vi "Dashboard Main.vi"() -> ()   [LabVIEW 2012]
uses:
  <vilib>/event_ctls.llb/eventvkey.ctl
  <vilib>/Utility/miscctls.llb/LVPointTypeDef.ctl
  <vilib>/Utility/config.llb/Read Key (String).vi
  <vilib>/Utility/config.llb/Read Key (I32).vi
  <vilib>/Utility/config.llb/Write Key (String).vi
  <vilib>/Utility/config.llb/Write Key (I32).vi
  <vilib>/Utility/config.llb/NI_LVConfig.lvlib
panel:
  in  "Camera Settings":T1={"Frate Rate"=30, "Compression"=51, "Size"=1} {"Frate Rate" scale=1.0..30.0; "Size" items=["640x480", "320x240", "160x120"]}
  out "Mode":T2(ring)=enum.""
  out "Camera IP":string="0.0.0.11"
  in  "Dashboard Tab":T3(tab)
  out "GO!! GO!! GO!!":bool
  out "Driver Ready":bool
  out "Shooter Speed":T4(ring)
  out "Shooter Encoder\nDead!!":bool
  out "Shooter Good":bool
  out "Dashboard Code Verzion":string
  out "Robot Code Version":string
  out "Shooter Good":bool
  out "Shooter Speed":dbl(graph)
  out "Wheel Speed":dbl
  out "Shooter Output":dbl
  out "Shooter Speed":T4(ring)
  out "Left Encoder":dbl
  out "Right Encoder":dbl
  out "Encoder Average":dbl
  out "Left Encoder Rate":dbl
  out "Right Encoder Rate":dbl
  out "Encoder Average Rate":dbl
  out "Gyro":dbl
  out "Battery Value":dbl(slide) scale=0.0..14.0 scale format="%#_2e"
  out "Battery":sgl(graph)
  out "JS1 Z":dbl(slide) scale=-1.0..1.0 scale format="%#_2e"
  out "JS2 Z":dbl(slide) scale=-1.0..1.0 scale format="%#_2e"
  out "Joystick 1":cluster{"X":dbl, "Y":dbl}[](graph)
  out "Joystick 2":cluster{"X":dbl, "Y":dbl}[](graph)
  out "JS Buttons 1":T5
  out "JS Buttons 2":T5
  out "MotorSlide4":dbl(slide) scale=-1.0..1.0 scale format="%#_2e"
  out "MotorSlide3":dbl(slide) scale=-1.0..1.0 scale format="%#_2e"
  out "MotorSlide2":dbl(slide) scale=-1.0..1.0 scale format="%#_2e"
  in  "MotorName3":string="Front Left"
  in  "MotorName4":string="Front Right"
  in  "MotorName1":string="Rear Left"
  in  "MotorName2":string="Rear Right"
  out "MotorChart4":dbl(graph)
  out "MotorChart3":dbl(graph)
  out "MotorChart2":dbl(graph)
  out "MotorSlide1":dbl(slide) scale=-1.0..1.0 scale format="%#_2e"
  out "MotorChart1":dbl(graph)
  out "Robot IP":string="0.0.0.0"
  in  "Slider":dbl(slide) scale=0.0..100.0 scale format="%#_3g"
  in  "On/Off":bool caption="Solenoid"
  in  "Test Name":u16(ring) items=["Select the test to run...", "Example Test", "-------------------------------", "List of tests is built in robot code.", "Replace with your own automated tests."]
  in  "Test Tree":string(tree)
  in  "Motor":cluster{"Value":dbl, "Enable":bool} {"Value" scale=-1.0..1.0 scale format="%#_3g"}
  out "Progress":T6 {"Test Progress" scale=0.0..100.0}
  in  "Rev/Fwd":cluster{"Forward":bool, "Reverse":bool}
  in  "Ring":u16(ring) items=["Auto", "Fixed indoor", "Fixed outdoor 1", "Fixed outdoor 2", "Fixed fluorescent 1", "Fixed fluorescent 2", "Hold current"]
  in  "Debug Mode":bool
  in  "Listbox":i32(listbox)
  in  "Viewer":T7(tab)
  in  "Enable Processing":bool=TRUE
  out "Mbps":dbl format="%#.1g"
  in  "Enable":bool=TRUE
  in  "DB Camera Config":bool
  out "Mbps":bool
  out "fps":dbl format="%#.1g"
  out "Image Error Message":string="Timeout in Camera Communications"
  out "Camera Image":T8(plugin-control)
  out "Vision Angle":dbl
  out "Buttons 1":cluster{"1":bool, "2":bool, "3":bool}
  out "Kinect 1":cluster{"X":dbl, "Y":dbl, "Z":dbl} {"X" scale=1.0..-1.0; "Y" scale=1.0..-1.0; "Z" scale=1.0..-1.0}
  out "Buttons 2":cluster{"1":bool, "2":bool, "3":bool}
  out "Kinect 2":cluster{"X":dbl, "Y":dbl, "Z":dbl} {"X" scale=1.0..-1.0; "Y" scale=1.0..-1.0; "Z" scale=1.0..-1.0}
  out "Version":string
  out "Skeleton Picture":picture
  out "Players":i8
  out "Tree":string(tree)
  # "Drive & Motors"
  # "Robot IP:"
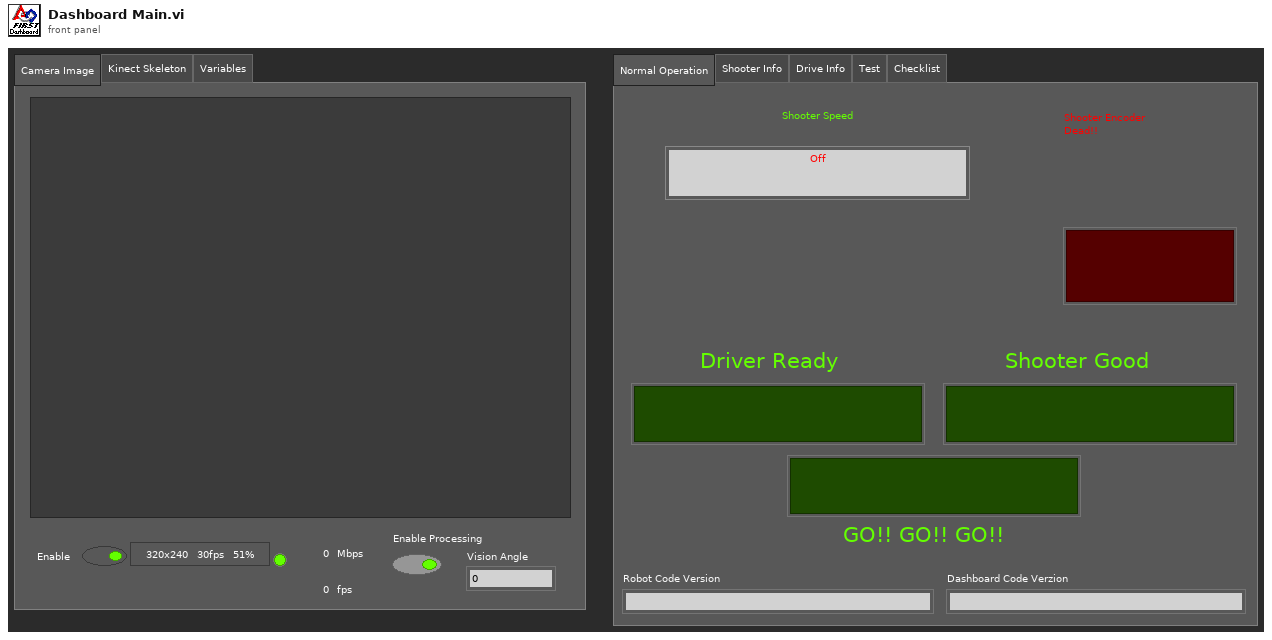
[diagram p1: front panel]
types:
  T1 = cluster{"Frate Rate":i32, "Compression":i32, "Size":u16}
  T2 = enum8{"Tele-Op Disabled", "Tele-Op Enabled", "Auto Disabled", "Auto Enabled", "Test Disabled", "Test Enabled", ""}
  T3 = enum32{"Normal Operation", "Shooter Info", "Drive Info", "Test", "Checklist"}
  T4 = enum16{"Off", "Close Pyramid 3pt", "Far Pyramid 3pt", "Feeder Shot", "UD Far 3pt Shot"}
  T5 = cluster{bool, bool, bool, bool, bool, bool, bool, bool, bool, bool, bool, bool}
  T6 = cluster{"Test Progress":u8, "Test Progress Text":string}
  T7 = enum32{"Camera Image", "Kinect Skeleton", "Variables"}
  T8 = typedef "IMAQ Image.ctl" = refnum<image>
  T9 = typedef "Image Type" = u32
  T10 = cluster{"Competition mode":bool, "Robot Link":bool, "Autonomous":bool, "Enabled":bool, "E-Stop":bool, "Simulated":bool, "TestMode":bool, "Docked Window":bool}
  T11 = cluster{"Boolean Array[0]":bool, "Boolean Array[1]":bool, "Boolean Array[2]":bool, "Boolean Array[3]":bool, "Boolean Array[4]":bool, "Boolean Array[5]":bool, "Boolean Array[6]":bool, "Boolean Array[7]":bool, "Boolean Array[8]":bool, "Boolean Array[9]":bool, "Boolean Array[10]":bool, "Boolean Array[11]":bool}
  T12 = typedef "LVPointTypeDef.ctl" = cluster{"Horizontal":i16, "Vertical":i16}
  T13 = typedef "LVRectTypeDef.ctl" = cluster{"Left":i16, "Top":i16, "Right":i16, "Bottom":i16}
  T14 = typedef "LVBoundsTypeDef.ctl" = cluster{"Width":u32, "Height":u32}
  T15 = typedef "SkeletonTrackState.ctl" = enum32{"NotTracked", "PositionOnly", "Tracked"}
  T16 = cluster{"TrackingState":u8[], "Position":cluster{"x":sgl, "y":sgl, "z":sgl}, cluster{"x":sgl, "y":sgl, "z":sgl, sgl}[], "TrackState":T15}
  T17 = cluster{cluster{"ScaledToPercentRange":dbl, "ScaledToPercentRange":dbl, "ScaledToPercentRange":dbl}, cluster{bool, bool, bool}}[]
  T18 = cluster{cluster{"ScaledToPercentRange":dbl, "ScaledToPercentRange":dbl, "ScaledToPercentRange":dbl}, cluster{bool, bool, bool}}
  T19 = cluster{"ScaledToPercentRange":dbl, "ScaledToPercentRange":dbl, "ScaledToPercentRange":dbl}
  T20 = typedef "NI_LVConfig.lvlib/Config Data RefNum.ctl" = refnum<k1>
  T21 = typedef "eventvkey.ctl" = enum16{"ASCII", "Enter", "Return", "Shift", "Ctrl", "Alt", "Cmd", "Opt", "Caps", "NumLock", "Clear", "Break", "Up", "Down", "Left", "Right", "Insert", "Delete", "Home", "End", "PageUp", "PageDown", "Escape", "Help", "Pause", "ScrollLock", "F1", "F2", "F3", "F4", "F5", "F6", "F7", "F8", "F9", "F10", "F11", "F12", "F13", "F14", "F15", "F16", "F17", "F18", "F19", "F20", "F21", "F22", "F23", "F24", "Play", "VolumeUp", "VolumeDown", "Mute", "Two Byte Char"}
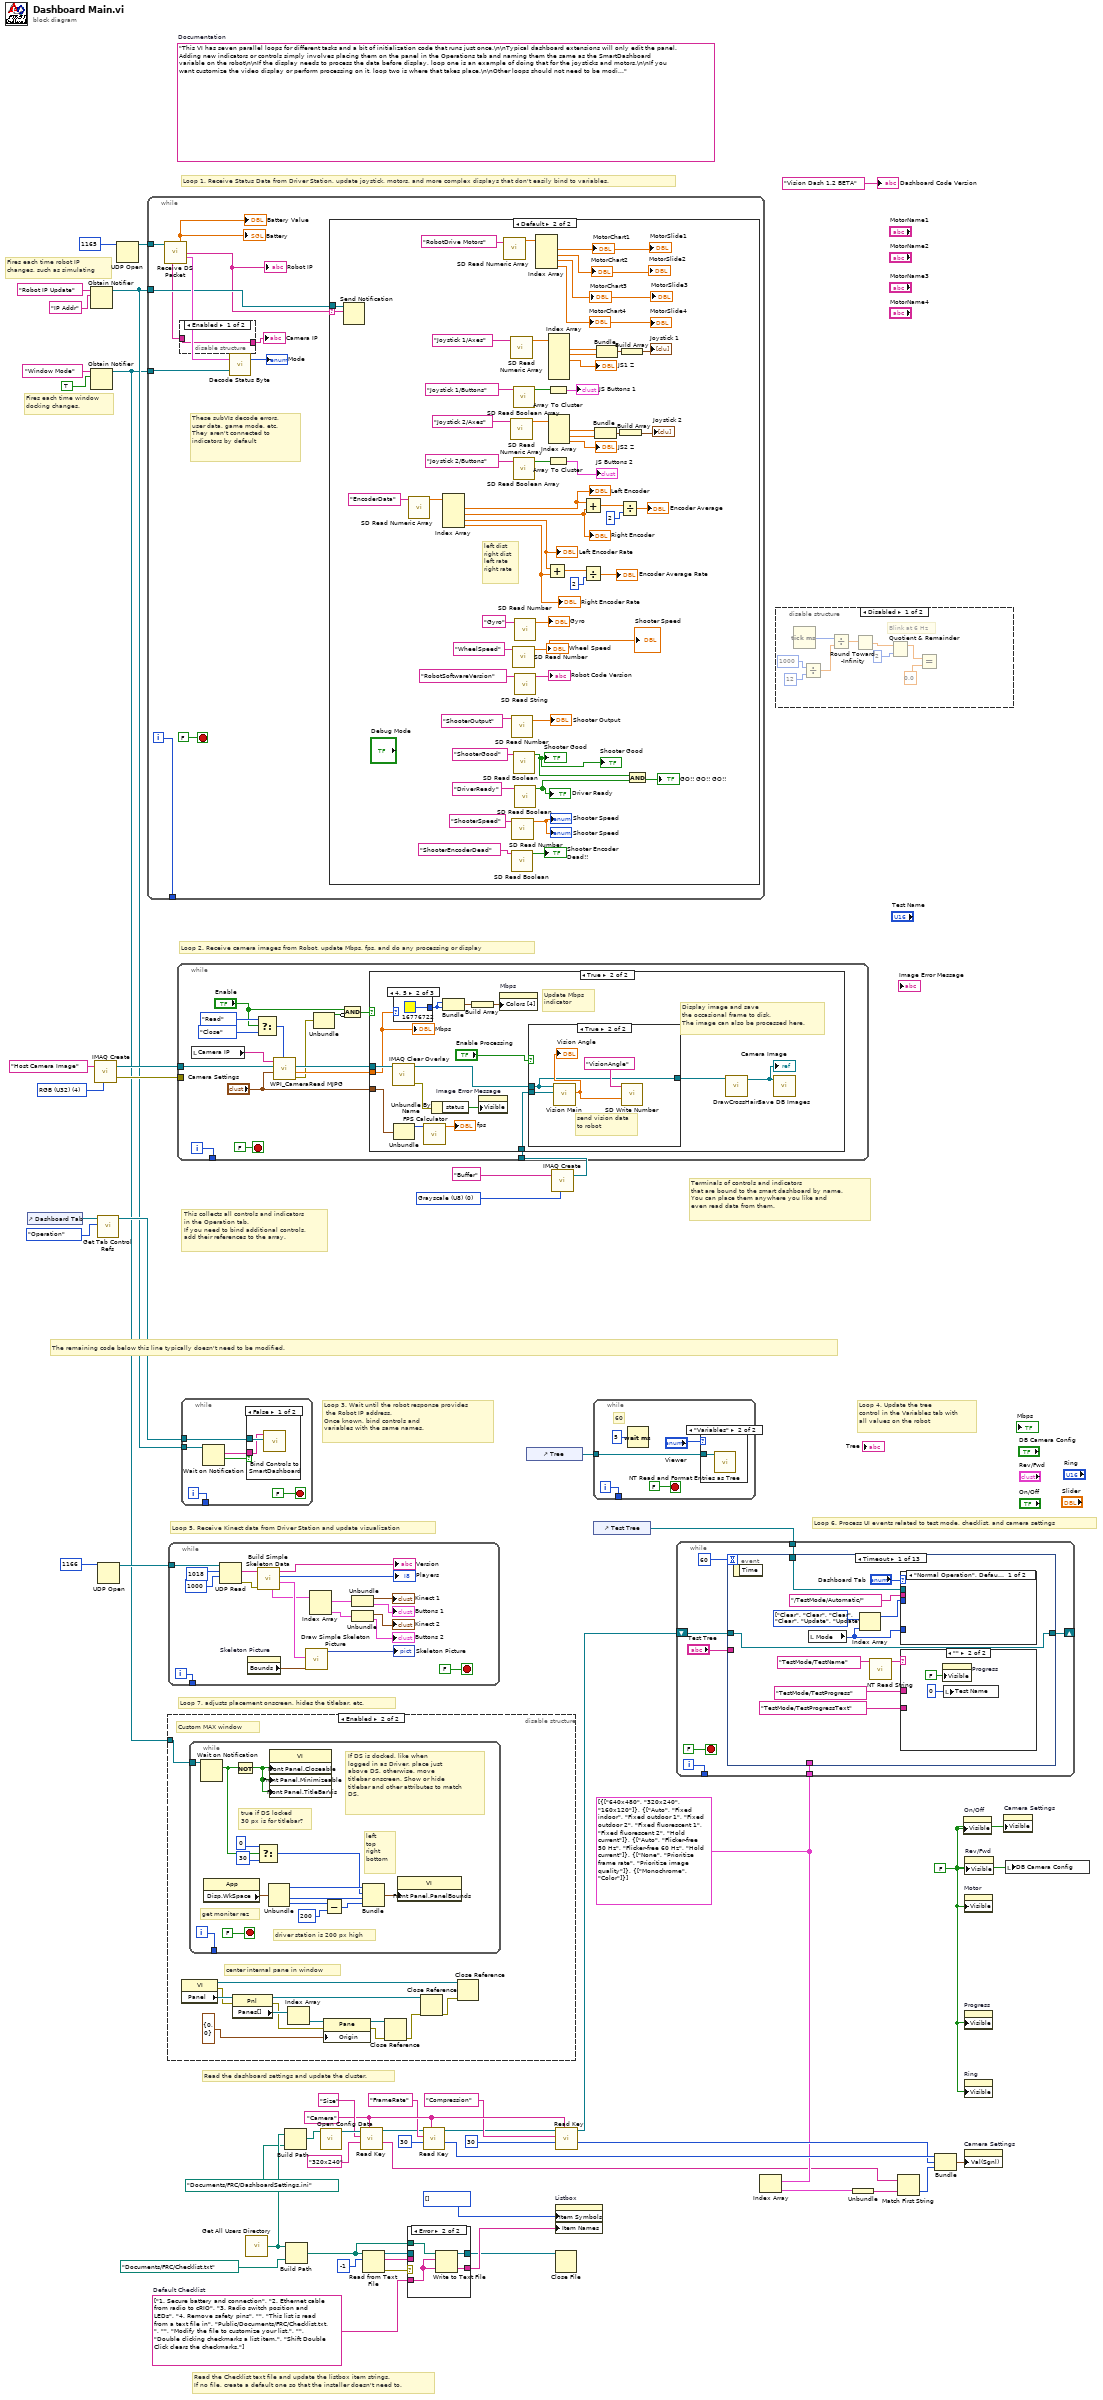
[diagram p0: block diagram]
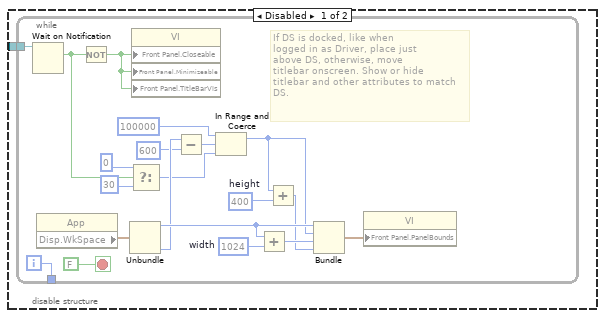
[diagram p3: hidden frame]
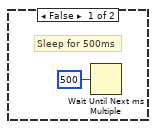
[diagram p5: hidden frame]
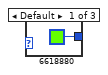
[diagram p7: hidden frame]
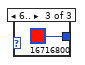
[diagram p8: hidden frame]
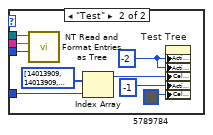
[diagram p10: hidden frame]
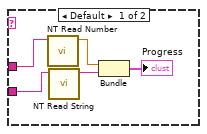
[diagram p11: hidden frame]
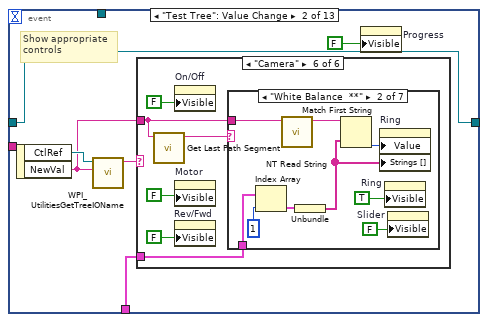
[diagram p12: hidden frame]
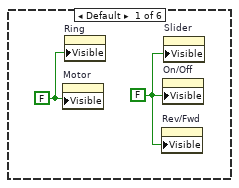
[diagram p13: hidden frame]
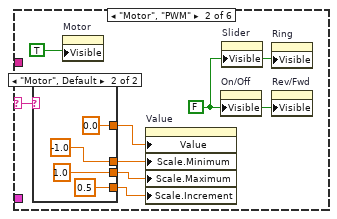
[diagram p14: hidden frame]
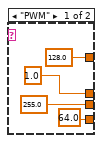
[diagram p15: hidden frame]
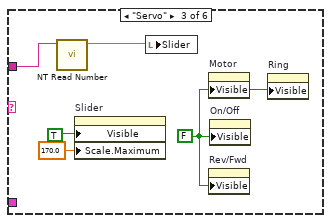
[diagram p16: hidden frame]
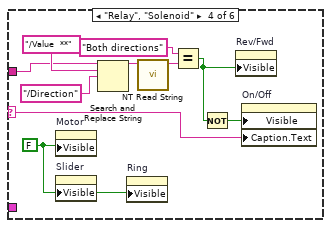
[diagram p17: hidden frame]
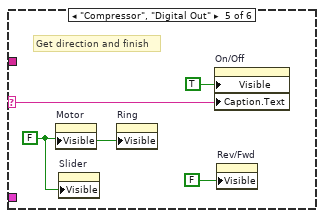
[diagram p18: hidden frame]
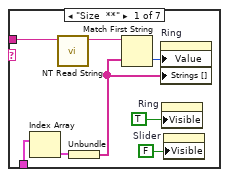
[diagram p19: hidden frame]
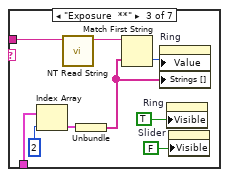
[diagram p20: hidden frame]
diagram:
  w3 = T9 0 items=["Grayscale (U8)", "Grayscale (I16)", "Grayscale (SGL)", "Complex (CSG)", "RGB (U32)", "HSL (U32)", "RGB (U64)", "Grayscale (U16)"] ("Image Type")
  w25 = "Camera"
  w17 = cluster{string[]}[] [{["640x480", "320x240", "160x120"]}, {["Auto", "Fixed indoor", "Fixed outdoor 1", "Fixed outdoor 2", "Fixed fluorescent 1", "Fixed fluorescent 2", "Hold current"]}, {["Auto", "Flicker-free 50 Hz", "Flicker-free 60 Hz", "Hold current"]}, {["None", "Prioritize frame rate", "Prioritize image quality"]}, {["Monochrome", "Color"]}]
  w33 = string[] ["1. Secure battery and connection", "2. Ethernet cable from radio to cRIO", "3. Radio switch position and LEDs", "4. Remove safety pins", "", "This list is read from a text file in", "Public/Documents/FRC/Checklist.txt.", "", "Modify the file to customize your list.", "", "Double clicking checkmarks a list item.", "Shift Double Click clears the checkmarks."]  # Default Checklist
  w31 = FALSE ("Visible")
  (unwired) "This VI has seven parallel loops for different tasks and a bit of initialization code that runs just once.\n\nTypical dashboard extensions will only edit the panel. Adding new indicators or controls simply involves placing them on the panel in the Operations tab and naming them the same as the SmartDashboard variable on the robot\n\nIf the display needs to process the data before display, loop one is an example of doing that for the joysticks and motors.\n\nIf you want customize the video display or perform processing on it, loop two is where that takes place.\n\nOther loops should not need to be modified. They are pretty standard, and document the task they perform."  # Documentation
  w54 = T9 4 items=["Grayscale (U8)", "Grayscale (I16)", "Grayscale (SGL)", "Complex (CSG)", "RGB (U32)", "HSL (U32)", "RGB (U64)"] ("Image Type")
  # "Fires each time robot IP\nchanges, such as simulating"
  # "Fires each time window\ndocking changes."
  # "Read the Checklist text file and update the listbox item strings.\nIf no file, create a default one so that the installer doesn't need to."
  # "This collects all controls and indicators\nin the Operation tab.\nIf you need to bind additional controls,\nadd their references to the array."
  # "The remaining code below this line typically doesn't need to be modified."
  # "Loop 6. Process UI events related to test mode, checklist, and camera settings"
  # "Read the dashboard settings and update the cluster."
  # "Terminals of controls and indicators\nthat are bound to the smart dashboard by name.\nYou can place them anywhere you like and\neven read data from them."
  # "Loop 4. Update the tree\ncontrol in the Variables tab with\nall values on the robot"
  # "Loop 3. Wait until the robot response provides\n the Robot IP address.\nOnce known, bind controls and\nvariables with the same names."
  # "Loop 5. Receive Kinect data from Driver Station and update visualization"
  # "Loop 7. adjusts placement onscreen, hides the titlebar, etc."
  # "Loop 1. Receive Status Data from Driver Station, update joystick, motors, and more complex displays that don't easily bind to variables."
  # "Loop 2. Receive camera images from Robot, update Mbps, fps, and do any processing or display"
  n1 = control-ref of="Dashboard Tab"() -> (w47:refnum<vi>)
  n2 = Obtain Notifier(name (unnamed)="Robot IP Update", notification data type="IP Addr" ("name (unnamed)")) -> (notifier out=w44:refnum<notifier>)  [unwired: 2 in, 2 out]
  n3 = Obtain Notifier(name (unnamed)="Window Mode", notification data type=TRUE) -> (notifier out=w37:refnum<notifier>)  [unwired: 2 in, 2 out]
  n4 = call "IMAQ Create"("Image Name"="Host Camera Image", "Image Type"=w54) -> ("New Image"=w52:T8, "error out"=w51:errorcluster)  [unwired: 2 in, 1 out]
  n5 = call <vilib>:"Get Tab Control Refs.vi"("Page Index"=enum32{"Operation", "Test"}."Operation" ("Dashboard Tab"), "TabControl in"=w47) -> ("ControlsOnPage"=w48:refnum<vi>[])  [unwired: 9 in]
  n6 = UDP Open(11:u16 1166 ("port")) -> (port=w49:refnum<k16>)  [unwired: 2 in, 4 out]
  n7 = UDP Open(11:u16 1165 ("port")) -> (port=w55:refnum<k16>)  [unwired: 2 in, 4 out]
  n8 = while {
    tunnel: w55 -> [w65]
    tunnel: w44 -> [w60]
    tunnel: w37 -> [w63]
    tunnel: [w61] -> _
    i -> [w61]
    stop <- FALSE stop-if-true
    # "These subVIs decode errors, user data, game mode, etc.\nThey aren't connected to indicators by default"
    n9 = call "Receive DS Packet.vi"("Recv Socket"=w65) -> ("Battery"=→"Battery" →"Battery Value":sgl, "Robot IP Address"=w59:string, "Status"=w66:T10, "Camera IP Address"=w57:string)  [unwired: 1 in, 10 out]
    "Robot IP" <- w59
    n10 = disable-structure shown="Enabled" {
      disable-tunnel: [w68 "10.16.76.11" ("Camera IP")] -> w58
      disable-tunnel: w57 -> [w68 _]
      frame Enabled {
      }
      frame Disabled {
      }
    }
    "Camera IP" <- w58
    n11 = call "Decode Status Byte.vi"("Window Mode Notifier"=w63, "Status"=w66) -> ("Mode"=→"Mode":T2)  [unwired: 1 out]
    n12 = case shown="Default" w59 {
      selector: w59 -> [_ w99]
      tunnel: w60 -> [_ w100]
      frame "0.0.0.0" {
        # "Robot not responding, don't poll the variables"
      }
      frame Default {
        # "left dist\nright dist\nleft rate\nright rate"
        n13 = Send Notification(notification=w99, notifier=w100) -> ()  [unwired: 1 in, 2 out]
        n14 = call <vilib>:"SD Read Numeric Array.vi"("Name"="EncoderData") -> ("Numeric Array"=w86:dbl[])  [unwired: 8 in, 2 out]
        n15 = Index Array(array=w86) -> (element #1=w85:dbl, element #2=w84:dbl, element #3=w80:dbl, element #4=w79:dbl)  [unwired: 4 in]
        "Left Encoder" <- w85
        "Right Encoder" <- w84
        "Left Encoder Rate" <- w80
        "Right Encoder Rate" <- w79
        n16 = call <vilib>:"SD Read Numeric Array.vi"("Name"="RobotDrive Motors") -> ("Numeric Array"=w123:dbl[])  [unwired: 8 in, 2 out]
        n17 = call <vilib>:"SD Read Numeric Array.vi"("Name"="Joystick 1/Axes") -> ("Numeric Array"=w116:dbl[])  [unwired: 8 in, 2 out]
        n18 = call <vilib>:"SD Read Numeric Array.vi"("Name"="Joystick 2/Axes") -> ("Numeric Array"=w110:dbl[])  [unwired: 8 in, 2 out]
        n19 = call <vilib>:"SD Read Number.vi"("Name"="ShooterOutput") -> ("Numeric"=→"Shooter Output":dbl)  [unwired: 8 in, 2 out]
        n20 = call <vilib>:"SD Read Boolean.vi"("Name"="ShooterEncoderDead") -> ("Boolean"=→"Shooter Encoder\nDead!!":bool)  [unwired: 8 in, 2 out]
        n21 = call <vilib>:"SD Read Number.vi"("Name"="ShooterSpeed") -> ("Numeric"=→"Shooter Speed" →"Shooter Speed":dbl)  [unwired: 8 in, 2 out]
        n22 = call <vilib>:"SD Read Number.vi"("Name"="WheelSpeed") -> ("Numeric"=→"Wheel Speed" →"Shooter Speed":dbl)  [unwired: 8 in, 2 out]
        n23 = call <vilib>:"SD Read Boolean Array.vi"("Name"="Joystick 1/Buttons") -> ("Boolean Array"=w118:bool[])  [unwired: 8 in, 2 out]
        n24 = call <vilib>:"SD Read Boolean Array.vi"("Name"="Joystick 2/Buttons") -> ("Boolean Array"=w109:bool[])  [unwired: 8 in, 2 out]
        n25 = call <vilib>:"SD Read Boolean.vi"("Name"="ShooterGood") -> ("Boolean"=w73:bool)  [unwired: 8 in, 2 out]
        "Shooter Good" <- w73
        "Shooter Good" <- w73
        n26 = call <vilib>:"SD Read Number.vi"("Name"="Gyro") -> ("Numeric"=→"Gyro":dbl)  [unwired: 8 in, 2 out]
        n27 = call <vilib>:"SD Read String.vi"("Name"="RobotSoftwareVersion") -> ("String"=→"Robot Code Version":string)  [unwired: 8 in, 2 out]
        n28 = call <vilib>:"SD Read Boolean.vi"("Name"="DriverReady") -> ("Boolean"=w72:bool)  [unwired: 8 in, 2 out]
        "Driver Ready" <- w72
        n29 = Index Array(array=w123) -> (element #1=→"MotorChart1" →"MotorSlide1":dbl, element #2=→"MotorSlide2" →"MotorChart2":dbl, element #3=→"MotorChart3" →"MotorSlide3":dbl, element #4=→"MotorChart4" →"MotorSlide4":dbl)  [unwired: 4 in]
        n30 = Add(x=w80, y=w79) -> (x+y=w81:dbl)
        n31 = Array To Cluster(array=w118) -> (cluster=→"JS Buttons 1":T11)
        n32 = Array To Cluster(array=w109) -> (cluster=→"JS Buttons 2":T11)
        n33 = Index Array(array=w116) -> (element #1=w113:dbl, element #2=w114:dbl, element #3=→"JS1 Z":dbl)  [unwired: 6 in, 3 out]
        n34 = Index Array(array=w110) -> (element #1=w105:dbl, element #2=w104:dbl, element #3=→"JS2 Z":dbl)  [unwired: 3 in]
        n35 = Add(x=w85, y=w84) -> (x+y=w95:dbl)
        n36 = Divide(x=w81, y=2) -> (x/y=→"Encoder Average Rate":dbl)
        n37 = Bundle("Numeric"=w105, "Numeric"=w104) -> (w106:cluster{"Numeric":dbl, "Numeric":dbl})  [unwired: 1 in]
        n38 = Bundle("Numeric"=w113, "Numeric"=w114) -> (w112:cluster{"Numeric":dbl, "Numeric":dbl})  [unwired: 1 in]
        n39 = Divide(x=w95, y=2) -> (x/y=→"Encoder Average":dbl)
        n40 = Build Array(w106) -> (→"Joystick 2":cluster{"Numeric":dbl, "Numeric":dbl}[])
        n41 = Build Array(w112) -> (→"Joystick 1":cluster{"Numeric":dbl, "Numeric":dbl}[])
        n42 = And(x=w73, y=w72) -> (x .and. y?=→"GO!! GO!! GO!!":bool)
      }
    }
  }
  n43 = disable-structure shown="Enabled" {
    disable-tunnel: w37 -> [w127 w160]
    frame Disabled {
      n44 = while {
        tunnel: w127 -> [w146]
        tunnel: [w144] -> _
        i -> [w144]
        stop <- FALSE stop-if-true
        w136 = 1024  # width
        w139 = 400  # height
        # "If DS is docked, like when\nlogged in as Driver, place just\nabove DS, otherwise, move\ntitlebar onscreen. Show or hide\ntitlebar and other attributes to match\nDS."
        n45 = Wait on Notification(notifier=w146) -> (notification=w131:bool)  [unwired: 3 in, 3 out]
        n46 = property class="App"() -> ("Disp.WkSpace"=w142:T13)  [unwired: 2 in, 2 out]
        n47 = Not(x=w131) -> (.not. x?=w145:bool)
        n48 = Unbundle(w142) -> ("Left"=w140:i16, "Bottom"=w137:i16)  [unwired: 2 out]
        n49 = Select(t=0, s=w131, f=30) -> (s? t:f=w130:i32)
        n50 = property class="VI"("Front Panel.Closeable"=w145, "Front Panel.Minimizeable"=w145, "Front Panel.TitleBarVis"=w145) -> ()  [unwired: 2 in, 2 out]
        n51 = Subtract(x=w137, y=600) -> (x-y=w134:i32)
        n52 = In Range and Coerce(upper limit=100000, x=w134, lower limit=w130) -> (coerced(x)=w128:i32)  [unwired: 1 out]
        n53 = Add(x=w140, y=w136) -> (x+y=w141:i32)
        n54 = Add(x=w128, y=w139) -> (x+y=w138:i32)
        n55 = Bundle("Left"=w140, w128, w141, w138) -> (w143:cluster{"Left":i16, i32, i32, i32})  [unwired: 1 out]
        n56 = property class="VI"("Front Panel.PanelBounds"=w143) -> ()  [unwired: 2 in, 2 out]
      }
    }
    frame Enabled {
      # "center internal pane in window"
      # "Custom MAX window"
      n57 = property class="VI"() -> (reference out=w153:refnum<vi>, error out=w152:errorcluster, "Panel"=w159:refnum<vi>)  [unwired: 2 in]
      n58 = while {
        tunnel: w160 -> [w174]
        tunnel: [w172] -> _
        i -> [w172]
        stop <- FALSE stop-if-true
        # "driver station is 200 px high"
        # "true if DS locked\n30 px is for titlebar?"
        # "left\ntop\nright\nbottom"
        # "get moniter rez"
        # "If DS is docked, like when\nlogged in as Driver, place just\nabove DS, otherwise, move\ntitlebar onscreen. Show or hide\ntitlebar and other attributes to match\nDS."
        n59 = Wait on Notification(notifier=w174) -> (notification=w166:bool)  [unwired: 3 in, 3 out]
        n60 = property class="App"() -> ("Disp.WkSpace"=w170:T13)  [unwired: 2 in, 2 out]
        n61 = Not(x=w166) -> (.not. x?=w173:bool)
        n62 = Select(t=0, s=w166, f=30) -> (s? t:f=w164:i32)
        n63 = Unbundle(w170) -> ("Left"=w169:i16, "Right"=w165:i16, "Bottom"=w162:i16)  [unwired: 1 out]
        n64 = property class="VI"("Front Panel.Closeable"=w173, "Front Panel.Minimizeable"=w173, "Front Panel.TitleBarVis"=w173) -> ()  [unwired: 2 in, 2 out]
        n65 = Subtract(x=w162, y=i16 200) -> (x-y=w163:i16)
        n66 = Bundle("Left"=w169, w164, "Right"=w165, w163) -> (w171:cluster{"Left":i16, i32, "Right":i16, i16})  [unwired: 1 out]
        n67 = property class="VI"("Front Panel.PanelBounds"=w171) -> ()  [unwired: 2 in, 2 out]
      }
      n68 = property class="Pnl"(reference=w159, error in=w152) -> (reference out=w154:refnum<vi>, error out=w151:errorcluster, "Panes[]"=w158:refnum<vi>[])
      n69 = Index Array(array=w158) -> (element=w157:refnum<vi>)  [unwired: 1 in]
      n70 = property class="Pane"(reference=w157, error in=w151, "Origin"=T12 {"Horizontal"=0, "Vertical"=0}) -> (reference out=w155:refnum<vi>, error out=w150:errorcluster)
      n71 = Close Reference(reference=w155, error in (no error)=w150) -> (error out=w149:errorcluster)
      n72 = Close Reference(reference=w154, error in (no error)=w149) -> (error out=w148:errorcluster)
      n73 = Close Reference(reference=w153, error in (no error)=w148) -> ()  [unwired: 1 out]
    }
  }
  n74 = while {
    tunnel: w49 -> [w192]
    tunnel: [w177] -> _
    i -> [w177]
    stop <- FALSE stop-if-true
    n75 = UDP Read(connection ID=w192, max size (548)=1018 ("bytes to read"), timeout ms (25000)=1000) -> (data out=w186:string, error out=w176:errorcluster)  [unwired: 1 in, 3 out]
    n76 = property on="Skeleton Picture" class="Pict"() -> ("Bounds"=w188:T14)  [unwired: 2 in, 2 out]
    n77 = call "Build Simple Skeleton Data.vi"("error in (no error)"=w176, "data in"=w186) -> ("Skeleton Data"=w187:T16, "NumPlayers"=→"Players":i8, "Version String"=→"Version":string, "Simple Joystick Info"=w184:T17)  [unwired: 5 in, 1 out]
    n78 = call "Draw Simple Skeleton Picture.vi"("Bounds"=w188, "Simple Skeleton"=w187) -> ("new picture out"=→"Skeleton Picture":picture)  [unwired: 9 in]
    n79 = Index Array(array=w184) -> (element #1=w183:T18, element #2=w182:T18)  [unwired: 2 in]
    n80 = Unbundle(w183) -> (→"Kinect 1":T19, →"Buttons 1":cluster{bool, bool, bool})
    n81 = Unbundle(w182) -> (→"Kinect 2":T19, →"Buttons 2":cluster{bool, bool, bool})
  }
  n82 = while {
    tunnel: w48 -> [w200]
    tunnel: w44 -> [w197]
    tunnel: [w195] -> _
    i -> [w195]
    stop <- FALSE stop-if-true
    n83 = Wait on Notification(notifier=w197) -> (notification=w196:string, timed out?=w198:bool)  [unwired: 3 in, 2 out]
    n84 = case shown="False" w198 {
      tunnel: w200 -> [w202 _]
      tunnel: w196 -> [w201 _]
      frame False {
        n85 = call <vilib>:"Bind Controls to SmartDashboard.vi"("Bound Control Refs"=w202, "Server IP Address"=w201) -> ()  [unwired: 10 in]
      }
      frame True {
      }
    }
  }
  n86 = call "Get All Users Directory.vi"() -> ("All User Path"=w30:path)
  n87 = Build Path(base path=w30, name or relative path=path "Documents/FRC/DashboardSettings.ini") -> (appended path=w29:path)
  n88 = Build Path(base path=w30, name or relative path=path "Documents/FRC/Checklist.txt") -> (appended path=w34:path)
  n89 = call <vilib>:"Open Config Data.vi"("configuration file path"=w29) -> ("refnum"=w28:T20)  [unwired: 8 in, 2 out]
  n90 = call-poly <vilib>:"Read Key.vi"("section"=w25, "default value"="320x240", "key"="Size", "refnum"=w28) -> ("value"=w15:string, "refnum out"=w10:T20)  [unwired: 2 in, 4 out]
  n91 = Read from Text File(file (use dialog)=w34, count=-1 ("timeout ms (25000)")) -> (refnum out=w12:refnum<file>, text=w35:string[], error out=w36:errorcluster)  [unwired: 2 in, 1 out]
  n92 = case shown="Error" w36 {
    tunnel: w35 -> [w204 _]
    tunnel: [w204 w206] -> w32
    tunnel: w33 -> [_ w206]
    tunnel: w34 -> [_ w207]
    tunnel: [w203 w205] -> w11
    tunnel: w12 -> [w203 _]
    frame No Error {
    }
    frame Error {
      n93 = Write to Text File(file (use dialog)=w207, text=w206) -> (refnum out=w205:refnum<file>)  [unwired: 2 in, 2 out]
    }
  }
  n94 = call-poly <vilib>:"Read Key.vi"("section"=w25, "default value"=30, "key"="FrameRate", "refnum"=w10) -> ("value"=w20:i32, "refnum out"=w9:T20)  [unwired: 1 in, 5 out]
  n95 = control-ref of="Tree"() -> (w6:refnum<vi>)
  n96 = call "IMAQ Create"("Image Name"="Buffer", "Image Type"=w3) -> ("New Image"=w2:T8)  [unwired: 3 in, 1 out]
  n97 = while {
    tunnel: w52 -> [w218]
    tunnel: w51 -> [_]
    tunnel: [w221] -> _
    tunnel: w2 -> [w208]
    i -> [w221]
    stop <- FALSE stop-if-true
    n98 = local read "Camera IP"() -> (w220:string)
    n99 = Select(t=enum16{"Read", "Reopen", "Close"}."Read" ("Operation"), s="Enable", f=enum16{"Read", "Reopen", "Close"}."Close" ("Operation")) -> (s? t:f=w213:enum16{"Read", "Reopen", "Close"})
    n100 = call <vilib>:"WPI_CameraRead MJPG.vi"("Operation"=w213, "Camera Settings"="Camera Settings", "Image"=w218, "address"=w220) -> ("error out"=w212:errorcluster, "Bandwidth (kbps)"=w216:dbl, "Image Out"=w217:T8)  [unwired: 5 in]
    n101 = Unbundle(w212) -> ("status"=w210:bool)  [unwired: 2 out]
    n102 = Compound Arithmetic op=AND("Enable", invert w210) -> (w209:bool)
    n103 = case shown="True" w209 {
      tunnel: "Camera Settings" -> [_ w230]
      tunnel: w217 -> [_ w233]
      tunnel: w216 -> [_ w232]
      tunnel: w208 -> [_ w228]
      frame False {
        # "Sleep for 500ms"
        n104 = Wait Until Next ms Multiple(millisecond multiple=u32 500) -> ()  [unwired: 1 out]
      }
      frame True {
        # "Display image and save\nthe occasional frame to disk.\nThe image can also be processed here."
        # "Update Mbps\nindicator"
        n105 = call "IMAQ Clear Overlay"("Image"=w233) -> ("error out"=w237:errorcluster, "Image Out"=w226:T8)  [unwired: 2 in, 7 out]
        n106 = case shown="4, 5" w232 {
          tunnel: [u32 6618880 ("Color Box") u32 16776722 ("Color Box") u32 16716800 ("Color Box")] -> w234
          frame Default {
          }
          frame 4, 5 {
          }
          frame 6.. {
          }
        }
        n107 = Unbundle(w230) -> ("Frate Rate"=w229:i32)  [unwired: 2 out]
        n108 = call "FPS Calculator.vi"("Average Count"=w229) -> ("fps"=→"fps":dbl)  [unwired: 10 in]
        n109 = Unbundle By Name(w237) -> ("status"=w238:bool)
        n110 = Bundle("Color Box"=w234, "Color Box"=w234) -> (w236:cluster{"Color Box":u32, "Color Box":u32})  [unwired: 1 out]
        n111 = Build Array(w236) -> (w235:cluster{"Color Box":u32, "Color Box":u32}[])
        n112 = property on="Image Error Message" class="Str"("Visible"=w238) -> ()  [unwired: 2 in, 2 out]
        n113 = property on="Mbps" class="Bool (strict)"("Colors [4]"=w235) -> ()  [unwired: 2 in, 2 out]
        n114 = case shown="True" "Enable Processing" {
          tunnel: w228 -> [_ w243]
          tunnel: w226 -> [w239 w240]
          tunnel: [w239 w240] -> w225
          frame False {
          }
          frame True {
            # "send vision data\nto robot"
            n115 = call "Vision Main.vi"("Frame Buffer"=w243, "Camera Image"=w240) -> ("Chosen Target Angle"=w241:dbl)  [unwired: 8 in, 1 out]
            "Vision Angle" <- w241
            n116 = call <vilib>:"SD Write Number.vi"("Numeric"=w241, "Name"="VisionAngle") -> ()  [unwired: 8 in, 2 out]
          }
        }
        n117 = call "DrawCrossHairs.vi"("Image In"=w225) -> ("Image Out"=w227:T8)  [unwired: 10 in]
        "Camera Image" <- w227
        n118 = call "Save DB Images.vi"("Image"=w227) -> ()  [unwired: 2 in, 1 out]
        "Mbps" <- w232
      }
    }
  }
  n119 = property on="Listbox" class="LstBox (strict)"("Item Symbols"=i32[] [], "Item Names"=w32) -> ()  [unwired: 2 in, 2 out]
  n120 = Close File(refnum=w11) -> ()  [unwired: 1 in, 2 out]
  n121 = call-poly <vilib>:"Read Key.vi"("section"=w25, "default value"=30, "key"="Compression", "refnum"=w9) -> ("value"=w19:i32, "refnum out"=w7:T20)  [unwired: 1 in, 5 out]
  n122 = while {
    tunnel: [w248] -> _
    tunnel: w6 -> [w247]
    i -> [w248]
    stop <- FALSE stop-if-true
    # "60"
    n123 = Wait (ms)(milliseconds to wait=u32 5) -> ()  [unwired: 1 out]
    n124 = case shown="\"Variables\"" "Viewer" {
      tunnel: w247 -> [_ w252]
      frame Default {
      }
      frame "Variables" {
        n125 = call <vilib>:"NT Read and Format Entries as Tree.vi"("Tree Refnum"=w252) -> ()  [unwired: 9 in, 2 out]
      }
    }
  }
  n126 = control-ref of="Test Tree"() -> (w5:refnum<vi>)
  n127 = while {
    tunnel: w17 -> [w257]
    shift-right: [w256] -> _
    shift-left: w7 -> [w255]
    tunnel: [w254] -> _
    tunnel: w5 -> [w253]
    i -> [w254]
    stop <- FALSE stop-if-true
    n128 = event shown="[0] Timeout" {
      selector: _ -> [_ _ _ _ _ _ _ _ _ _ _ _ _]
      dyn-events: _ -> [_ _ _ _ _ _ _ _ _ _ _ _ _]
      timeout: u32 60 ("milliseconds to wait") -> [_ _ _ _ _ _ _ _ _ _ _ _ _]
      tunnel: w253 -> [w267 _ _ _ _ _ _ _ _ _ _ _ _]
      tunnel: "Test Tree" -> [_ _ _ _ _ _ _ _ w461 w469 w471 w475 w483]
      tunnel: w257 -> [_ w289 _ _ _ _ w425 w455 _ _ _ _ _]
      tunnel: [w261 w288 _ w391 w399 w411 w424 w448 w460 w467 w470 w474 w482] -> w256
      tunnel: w255 -> [w261 w288 _ w391 w399 w411 w423 w448 w460 w467 w470 w474 w482]
      event Timeout {
        w266 = enum16{"Update", "Clear"}[] [enum."Clear", enum."Clear", enum."Clear", enum."Clear", enum."Update", enum."Update", enum."Clear"] items=["Update", "Clear"]
        n129 = event-data() -> ()  [unwired: 1 in, 1 out]
        n130 = local read "Mode"() -> (w264:T2)
        n131 = Index Array(array=w266, index=w264) -> (element=w265:enum16{"Update", "Clear"})
        n132 = call <vilib>:"NT Read String.vi"("Name"="TestMode/TestName") -> ("String"=w270:string)  [unwired: 9 in, 1 out]
        n133 = case shown="\"Normal Operation\", Default" "Dashboard Tab" {
          tunnel: w267 -> [_ w280]
          tunnel: "/TestMode/Automatic/" ("Name Pattern") -> [_ w279]
          tunnel: w265 -> [_ w278]
          tunnel: w264 -> [_ w276]
          frame "Normal Operation", Default {
          }
          frame "Test" {
            w275 = -2 ("Active Item:Row Number")
            n134 = call <vilib>:"NT Read and Format Entries as Tree.vi"("Operation"=w278, "Name Pattern"=w279, "Tree Refnum"=w280) -> ()  [unwired: 7 in, 2 out]
            n135 = Index Array(array=u32[] [14013909, 14013909, 14013909, 14013909, 14013909, 16777215, 14013909], index=w276) -> (element=w274:u32)
            n136 = property on="Test Tree" class="Tree (strict)"("Active Item Row Number"=w275, "ActiveColNum"=w275, "CellBG"=w274, "Active Item Row Number"=-1 ("Active Item:Row Number"), "CellBG"=u32 5789784 ("Color Box")) -> ()  [unwired: 2 in, 2 out]
          }
        }
        n137 = case shown="\"\"" w270 {
          tunnel: "TestMode/TestProgress" ("Name") -> [w282 _]
          tunnel: "TestMode/TestProgressText" ("Name") -> [w281 _]
          frame Default {
            n138 = call <vilib>:"NT Read Number.vi"("Name"=w282) -> ("Numeric"=w283:dbl)  [unwired: 9 in, 1 out]
            n139 = call <vilib>:"NT Read String.vi"("Name"=w281) -> ("String"=w284:string)  [unwired: 9 in, 1 out]
            n140 = Bundle("Numeric"=w283, "String"=w284) -> (→"Progress":cluster{"Numeric":dbl, "String":string})  [unwired: 1 in]
          }
          frame "" {
            n141 = property on="Progress" class="Clust (strict)"("Visible"=FALSE) -> ()  [unwired: 2 in, 2 out]
            n142 = local write "Test Name"(u16 0) -> ()
          }
        }
      }
      event "Test Tree": Value Change {
        # "Show appropriate\ncontrols"
        n143 = event-data() -> ("CtlRef"=w292:refnum<vi>, "NewVal"=w290:string)  [unwired: 1 in]
        n144 = call <vilib>:"WPI_UtilitiesGetTreeIOName.vi"("NewVal"=w290, "TreeControl in"=w292) -> ("I/O Name"=w293:string)  [unwired: 9 in]
        n145 = case shown="\"Camera\"" w293 {
          selector: w293 -> [_ w300 _ w318 w327 _]
          tunnel: w290 -> [_ _ w315 w317 _ w334]
          tunnel: w289 -> [_ _ _ _ _ w333]
          frame Default {
            w295 = FALSE ("Visible")
            w294 = FALSE ("Visible")
            n146 = property on="Motor" class="Clust (strict)"("Visible"=w294) -> ()  [unwired: 2 in, 2 out]
            n147 = property on="Ring" class="Ring (strict)"("Visible"=w294) -> ()  [unwired: 2 in, 2 out]
            n148 = property on="Rev/Fwd" class="Clust (strict)"("Visible"=w295) -> ()  [unwired: 2 in, 2 out]
            n149 = property on="On/Off" class="Bool (strict)"("Visible"=w295) -> ()  [unwired: 2 in, 2 out]
            n150 = property on="Slider" class="Slide (strict)"("Visible"=w295) -> ()  [unwired: 2 in, 2 out]
          }
          frame "Motor", "PWM" {
            w301 = FALSE ("Visible")
            n151 = case shown="\"Motor\", Default" w300 {
              tunnel: [1.0 ("Value") -1.0 ("Value")] -> w299
              tunnel: [255.0 ("Value") 1.0 ("Value")] -> w298
              tunnel: [128.0 ("Value") 0.0 ("Value")] -> w297
              tunnel: [64.0 ("Value") 0.5 ("Value")] -> w296
              frame "PWM" {
              }
              frame "Motor", Default {
              }
            }
            n152 = property on="Motor" class="Clust (strict)"("Visible"=TRUE) -> ()  [unwired: 2 in, 2 out]
            n153 = property on="Value" class="Slide (strict)"("Value"=w297, "Scale.Minimum"=w299, "Scale.Maximum"=w298, "Scale.Increment"=w296) -> ()  [unwired: 2 in, 2 out]
            n154 = property on="On/Off" class="Bool (strict)"("Visible"=w301) -> ()  [unwired: 2 in, 2 out]
            n155 = property on="Slider" class="Slide (strict)"("Visible"=w301) -> ()  [unwired: 2 in, 2 out]
            n156 = property on="Ring" class="Ring (strict)"("Visible"=w301) -> ()  [unwired: 2 in, 2 out]
            n157 = property on="Rev/Fwd" class="Clust (strict)"("Visible"=w301) -> ()  [unwired: 2 in, 2 out]
          }
          frame "Servo" {
            w313 = FALSE ("Visible")
            n158 = call <vilib>:"NT Read Number.vi"("Name"=w315) -> ("Numeric"=w314:dbl)  [unwired: 9 in, 1 out]
            n159 = property on="Slider" class="Slide (strict)"("Visible"=TRUE, "Scale.Maximum"=170.0 ("Scale.Range:Maximum")) -> ()  [unwired: 2 in, 2 out]
            n160 = local write "Slider"(w314) -> ()
            n161 = property on="Motor" class="Clust (strict)"("Visible"=w313) -> ()  [unwired: 2 in, 2 out]
            n162 = property on="Rev/Fwd" class="Clust (strict)"("Visible"=w313) -> ()  [unwired: 2 in, 2 out]
            n163 = property on="On/Off" class="Bool (strict)"("Visible"=w313) -> ()  [unwired: 2 in, 2 out]
            n164 = property on="Ring" class="Ring (strict)"("Visible"=w313) -> ()  [unwired: 2 in, 2 out]
          }
          frame "Relay", "Solenoid" {
            w316 = FALSE ("Visible")
            n165 = property on="Motor" class="Clust (strict)"("Visible"=w316) -> ()  [unwired: 2 in, 2 out]
            n166 = property on="Slider" class="Slide (strict)"("Visible"=w316) -> ()  [unwired: 2 in, 2 out]
            n167 = Search and Replace String(input string=w317, search string="/Value  **", replace string="/Direction") -> (result string=w323:string)  [unwired: 5 in, 3 out]
            n168 = property on="Ring" class="Ring (strict)"("Visible"=w316) -> ()  [unwired: 2 in, 2 out]
            n169 = call <vilib>:"NT Read String.vi"("Name"=w323) -> ("String"=w321:string)  [unwired: 9 in, 1 out]
            n170 = Equal?(x="Both directions", y=w321) -> (x = y?=w319:bool)
            n171 = Not(x=w319) -> (.not. x?=w320:bool)
            n172 = property on="Rev/Fwd" class="Clust (strict)"("Visible"=w319) -> ()  [unwired: 2 in, 2 out]
            n173 = property on="On/Off" class="Bool (strict)"("Visible"=w320, "Caption.Text"=w318) -> ()  [unwired: 2 in, 2 out]
          }
          frame "Compressor", "Digital Out" {
            w326 = FALSE ("Visible")
            # "Get direction and finish"
            n174 = property on="Motor" class="Clust (strict)"("Visible"=w326) -> ()  [unwired: 2 in, 2 out]
            n175 = property on="Slider" class="Slide (strict)"("Visible"=w326) -> ()  [unwired: 2 in, 2 out]
            n176 = property on="Ring" class="Ring (strict)"("Visible"=w326) -> ()  [unwired: 2 in, 2 out]
            n177 = property on="On/Off" class="Bool (strict)"("Visible"=TRUE, "Caption.Text"=w327) -> ()  [unwired: 2 in, 2 out]
            n178 = property on="Rev/Fwd" class="Clust (strict)"("Visible"=FALSE) -> ()  [unwired: 2 in, 2 out]
          }
          frame "Camera" {
            n179 = call <vilib>:"Get Last Path Segment.vi"("String in"=w334) -> ("String out"=w335:string)  [unwired: 10 in]
            n180 = property on="On/Off" class="Bool (strict)"("Visible"=FALSE) -> ()  [unwired: 2 in, 2 out]
            n181 = property on="Motor" class="Clust (strict)"("Visible"=FALSE) -> ()  [unwired: 2 in, 2 out]
            n182 = property on="Rev/Fwd" class="Clust (strict)"("Visible"=FALSE) -> ()  [unwired: 2 in, 2 out]
            n183 = case shown="\"White Balance  **\"" w335 {
              tunnel: w334 -> [w341 w350 w359 w368 w377 _ w383]
              tunnel: w333 -> [w339 w347 w356 w365 w374 _ _]
              frame "Size  **" {
                n184 = Index Array(array=w339) -> (element=w338:cluster{string[]})  [unwired: 1 in]
                n185 = call <vilib>:"NT Read String.vi"("Name"=w341) -> ("String"=w340:string)  [unwired: 9 in, 1 out]
                n186 = Unbundle(w338) -> (w336:string[])
                n187 = Match First String(2:w336, 3:w340) -> (0:w337:i32)  [unwired: 1 out]
                n188 = property on="Ring" class="Ring (strict)"("Value"=w337, "Strings []"=w336) -> ()  [unwired: 2 in, 2 out]
                n189 = property on="Ring" class="Ring (strict)"("Visible"=TRUE) -> ()  [unwired: 2 in, 2 out]
                n190 = property on="Slider" class="Slide (strict)"("Visible"=FALSE) -> ()  [unwired: 2 in, 2 out]
              }
              frame "White Balance  **" {
                n191 = Index Array(array=w347, index=1) -> (element=w348:cluster{string[]})
                n192 = call <vilib>:"NT Read String.vi"("Name"=w350) -> ("String"=w349:string)  [unwired: 9 in, 1 out]
                n193 = Unbundle(w348) -> (w345:string[])
                n194 = Match First String(2:w345, 3:w349) -> (0:w344:i32)  [unwired: 1 out]
                n195 = property on="Ring" class="Ring (strict)"("Value"=w344, "Strings []"=w345) -> ()  [unwired: 2 in, 2 out]
                n196 = property on="Ring" class="Ring (strict)"("Visible"=TRUE) -> ()  [unwired: 2 in, 2 out]
                n197 = property on="Slider" class="Slide (strict)"("Visible"=FALSE) -> ()  [unwired: 2 in, 2 out]
              }
              frame "Exposure  **" {
                n198 = Index Array(array=w356, index=2) -> (element=w357:cluster{string[]})
                n199 = call <vilib>:"NT Read String.vi"("Name"=w359) -> ("String"=w358:string)  [unwired: 9 in, 1 out]
                n200 = Unbundle(w357) -> (w353:string[])
                n201 = Match First String(2:w353, 3:w358) -> (0:w354:i32)  [unwired: 1 out]
                n202 = property on="Ring" class="Ring (strict)"("Value"=w354, "Strings []"=w353) -> ()  [unwired: 2 in, 2 out]
                n203 = property on="Ring" class="Ring (strict)"("Visible"=TRUE) -> ()  [unwired: 2 in, 2 out]
                n204 = property on="Slider" class="Slide (strict)"("Visible"=FALSE) -> ()  [unwired: 2 in, 2 out]
              }
              frame "Exposure Priority  **" {
                n205 = Index Array(array=w365, index=3) -> (element=w366:cluster{string[]})
                n206 = call <vilib>:"NT Read String.vi"("Name"=w368) -> ("String"=w367:string)  [unwired: 9 in, 1 out]
                n207 = Unbundle(w366) -> (w362:string[])
                n208 = Match First String(2:w362, 3:w367) -> (0:w363:i32)  [unwired: 1 out]
                n209 = property on="Ring" class="Ring (strict)"("Value"=w363, "Strings []"=w362) -> ()  [unwired: 2 in, 2 out]
                n210 = property on="Ring" class="Ring (strict)"("Visible"=TRUE) -> ()  [unwired: 2 in, 2 out]
                n211 = property on="Slider" class="Slide (strict)"("Visible"=FALSE) -> ()  [unwired: 2 in, 2 out]
              }
              frame "Color Enable  **" {
                n212 = Index Array(array=w374, index=4) -> (element=w375:cluster{string[]})
                n213 = call <vilib>:"NT Read String.vi"("Name"=w377) -> ("String"=w376:string)  [unwired: 9 in, 1 out]
                n214 = Unbundle(w375) -> (w371:string[])
                n215 = Match First String(2:w371, 3:w376) -> (0:w372:i32)  [unwired: 1 out]
                n216 = property on="Ring" class="Ring (strict)"("Value"=w372, "Strings []"=w371) -> ()  [unwired: 2 in, 2 out]
                n217 = property on="Ring" class="Ring (strict)"("Visible"=TRUE) -> ()  [unwired: 2 in, 2 out]
                n218 = property on="Slider" class="Slide (strict)"("Visible"=FALSE) -> ()  [unwired: 2 in, 2 out]
              }
              frame Default {
                n219 = property on="Ring" class="Ring (strict)"("Visible"=FALSE) -> ()  [unwired: 2 in, 2 out]
                n220 = property on="Slider" class="Slide (strict)"("Visible"=FALSE) -> ()  [unwired: 2 in, 2 out]
              }
              frame "Brightness  **", "Color Level  **", "Compression  **", "FPS  **", "Sharpness  **" {
                n221 = call <vilib>:"NT Read Number.vi"("Name"=w383) -> ("Numeric"=w382:dbl)  [unwired: 9 in, 1 out]
                n222 = local write "Slider"(w382) -> ()
                n223 = property on="Slider" class="Slide (strict)"("Visible"=TRUE, "Scale.Maximum"=100.0 ("Scale.Range:Maximum")) -> ()  [unwired: 2 in, 2 out]
                n224 = property on="Ring" class="Ring (strict)"("Visible"=FALSE) -> ()  [unwired: 2 in, 2 out]
              }
            }
          }
        }
        n225 = property on="Progress" class="Clust (strict)"("Visible"=FALSE) -> ()  [unwired: 2 in, 2 out]
      }
      event "Test Name": Mouse Enter {
        # "Populate the ring with the list of tests"
        n226 = event-data() -> ()  [unwired: 1 in, 1 out]
        n227 = call <vilib>:"NT Read String Array.vi"("Name"="TestMode/TestList") -> ("String Array"=w390:string[])  [unwired: 9 in, 1 out]
        n228 = Build Array (concatenate)("Select the test to run...", w390) -> (w389:string[])
        n229 = property on="Test Name" class="Ring (strict)"("Strings []"=w389) -> ()  [unwired: 2 in, 2 out]
      }
      event "Test Name": Value Change {
        w392 = FALSE ("Visible")
        # "Tell the robot the test name to run"
        n230 = event-data() -> ("NewVal"=w396:u16)  [unwired: 1 in]
        n231 = property on="Test Name" class="Ring (strict)"() -> ("Strings []"=w397:string[])  [unwired: 2 in, 2 out]
        n232 = local write "Progress"(T6 {"Test Progress"=0, "Test Progress Text"=""} ("Progress")) -> ()
        n233 = Index Array(array=w397, index=w396) -> (element=w395:string)
        n234 = call <vilib>:"NT Write String.vi"("String"=w395, "Name"="TestMode/TestName") -> ()  [unwired: 9 in, 1 out]
        n235 = property on="Progress" class="Clust (strict)"("Visible"=TRUE) -> ()  [unwired: 2 in, 2 out]
        n236 = property on="Motor" class="Clust (strict)"("Visible"=w392) -> ()  [unwired: 2 in, 2 out]
        n237 = property on="Slider" class="Slide (strict)"("Visible"=w392) -> ()  [unwired: 2 in, 2 out]
        n238 = property on="On/Off" class="Bool (strict)"("Visible"=w392) -> ()  [unwired: 2 in, 2 out]
        n239 = property on="Rev/Fwd" class="Clust (strict)"("Visible"=w392) -> ()  [unwired: 2 in, 2 out]
        n240 = property on="Ring" class="Ring (strict)"("Visible"=w392) -> ()  [unwired: 2 in, 2 out]
      }
      event "Listbox": Double Click {
        n241 = event-data() -> ("PlatMods.Shift"=w400:bool, "Row"=w402:i32)  [unwired: 1 in]
        n242 = case shown="False" w400 {
          tunnel: w402 -> [w406 _]
          tunnel: 1 -> [w405 _]
          frame False {
            n243 = property on="Listbox" class="LstBox (strict)"() -> ("Item Symbols"=w404:i32[])  [unwired: 2 in, 2 out]
            n244 = Replace Array Subset(array=w404, new element=w405, index=w406) -> (w403:i32[])
            n245 = property on="Listbox" class="LstBox (strict)"("Item Symbols"=w403) -> ()  [unwired: 2 in, 2 out]
          }
          frame True {
            w407 = 0 ("Top Row")
            n246 = property on="Listbox" class="LstBox (strict)"() -> ("Number of Rows"=w409:u32)  [unwired: 2 in, 2 out]
            n247 = Initialize Array(0, w409) -> (w408:i32[])
            n248 = property on="Listbox" class="LstBox (strict)"("Top Row"=w407, "Value"=w407, "Item Symbols"=w408) -> ()  [unwired: 2 in, 2 out]
          }
        }
      }
      event "Listbox": Key Down {
        n249 = event-data() -> ("VKey"=w413:T21)  [unwired: 1 in]
        n250 = case shown="\"Left\", \"Right\"" w413 {
          selector: w413 -> [w418 _]
          tunnel: eventvkey."Left" ("VKey") -> [w416 _]
          frame "Left", "Right" {
            n251 = Equal?(x=w416, y=w418) -> (x = y?=w417:bool)
            n252 = Select(t=0, s=w417, f=1) -> (s? t:f=w419:i32)
            n253 = property on="Listbox" class="LstBox (strict)"() -> ("Item Symbols"=w422:i32[])  [unwired: 2 in, 2 out]
            n254 = Replace Array Subset(array=w422, new element=w419, index="Listbox") -> (w421:i32[])
            n255 = property on="Listbox" class="LstBox (strict)"("Item Symbols"=w421) -> ()  [unwired: 2 in, 2 out]
          }
          frame Default {
          }
        }
      }
      event "DB Camera Config": Value Change {
        n256 = event-data() -> ("NewVal"=w426:bool)  [unwired: 1 in]
        n257 = case shown="False" w426 {
          tunnel: w425 -> [w435 _]
          tunnel: [w428 w446] -> w424
          tunnel: w423 -> [w427 w446]
          frame False {
            w442 = "Camera"
            w445 = FALSE ("Visible")
            n258 = local read "Camera Settings"() -> (w434:T1)
            n259 = Index Array(array=w435) -> (element=w438:cluster{string[]})  [unwired: 1 in]
            n260 = Unbundle(w434) -> ("Frate Rate"=w433:i32, "Compression"=w432:i32, "Size"=w436:u16)
            n261 = Unbundle(w438) -> (w437:string[])
            n262 = Index Array(array=w437, index=w436) -> (element=w431:string)
            n263 = call-poly <vilib>:"Write Key.vi"("section"=w442, "value"=w431, "key"="Size", "refnum"=w427) -> ("refnum out"=w444:T20)  [unwired: 2 in, 5 out]
            n264 = call-poly <vilib>:"Write Key.vi"("section"=w442, "value"=w433, "key"="FrameRate", "refnum"=w444) -> ("refnum out"=w443:T20)  [unwired: 1 in, 6 out]
            n265 = property on="Camera Settings" class="Clust (strict)"("Visible"=w445) -> ()  [unwired: 2 in, 2 out]
            n266 = local write "DB Camera Config"(w445) -> ()
            n267 = call-poly <vilib>:"Write Key.vi"("section"=w442, "value"=w432, "key"="Compression", "refnum"=w443) -> ("refnum out"=w429:T20)  [unwired: 1 in, 6 out]
            n268 = call <vilib>:"Close Config Data.vi"("refnum"=w429) -> ("file path"=w430:path)  [unwired: 2 in, 8 out]
            n269 = call <vilib>:"Open Config Data.vi"("configuration file path"=w430) -> ("refnum"=w428:T20)  [unwired: 8 in, 2 out]
          }
          frame True {
            n270 = property on="Camera Settings" class="Clust (strict)"("Visible"=TRUE) -> ()  [unwired: 2 in, 2 out]
          }
        }
      }
      event "Camera Settings": Value Change {
        n271 = event-data() -> ("NewVal"=w459:T1)  [unwired: 1 in]
        n272 = Index Array(array=w455) -> (element=w454:cluster{string[]})  [unwired: 1 in]
        n273 = Unbundle(w459) -> ("Frate Rate"=w450:i32, "Compression"=w449:i32, "Size"=w452:u16)
        n274 = Unbundle(w454) -> (w453:string[])
        n275 = Index Array(array=w453, index=w452) -> (element=w451:string)
        n276 = Format Into String(format string="%s   %dfps   %d%%", w451, w450, w449) -> (resulting string=w456:string)  [unwired: 2 in, 1 out]
        n277 = Build Array(w456) -> (w457:string[])
        n278 = property on="DB Camera Config" class="Bool (strict)"("Strings [4]"=w457) -> ()  [unwired: 2 in, 2 out]
      }
      event "Motor.Enable": Value Change {
        n279 = event-data() -> ("NewVal"=w465:bool)  [unwired: 1 in]
        n280 = Unbundle("Motor") -> ("Value"=w464:dbl)  [unwired: 1 out]
        n281 = Select(t=w464, s=w465, f=0.0) -> (s? t:f=w462:dbl)
        n282 = call <vilib>:"NT Write Number.vi"("Numeric"=w462, "Name"=w461) -> ()  [unwired: 9 in, 1 out]
      }
      event "Slider": Value Change {
        n283 = event-data() -> ("NewVal"=w468:dbl)  [unwired: 1 in]
        n284 = call <vilib>:"NT Write Number.vi"("Numeric"=w468, "Name"=w469) -> ()  [unwired: 9 in, 1 out]
      }
      event "On/Off": Value Change {
        n285 = event-data() -> ("NewVal"=w473:bool)  [unwired: 1 in]
        n286 = Boolean To (0,1)(Boolean=w473) -> (0, 1=w472:i16)
        n287 = call <vilib>:"NT Write Number.vi"("Numeric"=w472, "Name"=w471) -> ()  [unwired: 9 in, 1 out]
      }
      event "Rev/Fwd": Value Change {
        n288 = event-data() -> ("NewVal.Forward"=w481:bool, "NewVal.Reverse"=w480:bool)  [unwired: 1 in]
        n289 = Boolean To (0,1)(Boolean=w481) -> (0, 1=w477:i16)
        n290 = Boolean To (0,1)(Boolean=w480) -> (0, 1=w479:i16)
        n291 = Negate(x=w479) -> (-x=w478:i16)
        n292 = Add(x=w477, y=w478) -> (x+y=w476:i16)
        n293 = call <vilib>:"NT Write Number.vi"("Numeric"=w476, "Name"=w475) -> ()  [unwired: 9 in, 1 out]
      }
      event "Ring": Value Change {
        n294 = event-data() -> ("NewVal"=w485:u16)  [unwired: 1 in]
        n295 = property on="Ring" class="Ring (strict)"() -> ("Strings []"=w486:string[])  [unwired: 2 in, 2 out]
        n296 = Index Array(array=w486, index=w485) -> (element=w484:string)
        n297 = call <vilib>:"NT Write String.vi"("String"=w484, "Name"=w483) -> ()  [unwired: 9 in, 1 out]
      }
    }
  }
  n298 = Index Array(array=w17) -> (element=w18:cluster{string[]})  [unwired: 1 in]
  n299 = disable-structure shown="Disabled" {
    frame Disabled {
      # "Blink at 6 Hz"
      n300 = Tick Count (ms)() -> (millisecond timer value=w487:u32)
      n301 = Divide(x=1000, y=12) -> (x/y=w490:dbl)
      n302 = Divide(x=w487, y=w490) -> (x/y=w492:dbl)
      n303 = Round Toward -Infinity(1:w492) -> (0:w493:dbl)
      n304 = Quotient & Remainder(x=w493, y=2) -> (x-y*floor(x/y)=w494:dbl)  [unwired: 1 out]
      n305 = Equal?(x=w494, y=0.0) -> (x = y?=w496:bool)
    }
    frame Enabled {
    }
  }
  n306 = Unbundle(w18) -> (w16:string[])
  n307 = Match First String(2:w16, 3:w15) -> (0:w14:i32)  [unwired: 1 out]
  n308 = Bundle("value"=w20, "value"=w19, "index"=w14) -> (w8:cluster{"value":i32, "value":i32, "index":i32})  [unwired: 1 out]
  n309 = property on="On/Off" class="Bool (strict)"("Visible"=w31) -> ()  [unwired: 2 in, 2 out]
  n310 = property on="Motor" class="Clust (strict)"("Visible"=w31) -> ()  [unwired: 2 in, 2 out]
  n311 = property on="Progress" class="Clust (strict)"("Visible"=w31) -> ()  [unwired: 2 in, 2 out]
  n312 = property on="Ring" class="Ring (strict)"("Visible"=w31) -> ()  [unwired: 2 in, 2 out]
  n313 = property on="Camera Settings" class="Clust (strict)"("Val(Sgnl)"=w8) -> ()  [unwired: 2 in, 2 out]
  n314 = property on="Rev/Fwd" class="Clust (strict)"("Visible"=w31) -> ()  [unwired: 2 in, 2 out]
  n315 = property on="Camera Settings" class="Clust (strict)"("Visible"=w31) -> ()  [unwired: 2 in, 2 out]
  n316 = local write "DB Camera Config"(w31) -> ()
  "Dashboard Code Verzion" <- "Vision Dash 1.2 BETA" ("Dashboard Code Verzion")
